vi "Execute_SQL.vi"(6 "commandTimeout in":i32=-1, 7 "CommandType":i32(ring)=-1 items=["Text"=1, "StoredProcedure"=4, "TableDirect"=512], 8 "error in (no error)":errorcluster, 9 "Parameters In":variant, 10 "sql":string, 11 "SqlMapper in":refnum<class "SqlMapper.lvclass">) -> (0 "error out":errorcluster, 1 "affectedRows":i32, 3 "SqlMapper out":refnum<class "SqlMapper.lvclass">)   [LabVIEW 2020, in "ORM_API.lvlib"]
uses:
  ORM_API.lvlib
  <vilib>/Viviota/shared/ORM.lvlibp/ORM/SqlMapper/SqlMapper.lvclass
  <vilib>/Viviota/shared/ORM.lvlibp/ORM/TypeMap/Create DynamicParameter.vi
  <vilib>/Viviota/shared/ORM.lvlibp/ORM/DynamicParameters/DynamicParameters.lvclass
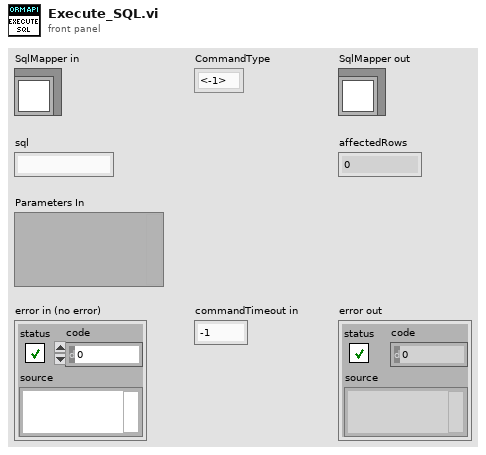
[diagram p1: front panel]
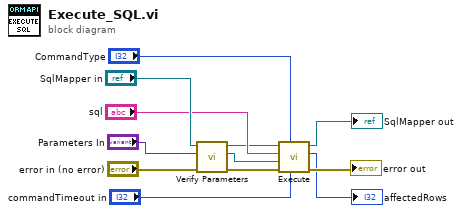
[diagram p0: block diagram]
diagram:
  n1 = call "Verify Parameters.vi"("error in (no error)"="error in (no error)", "Parameters In"="Parameters In", "SqlMapper in"="SqlMapper in") -> ("error out"=w7:errorcluster, "DynamicParameters out"=w6:refnum<class "DynamicParameters.lvclass">, "SqlMapper out"=w4:refnum<class "SqlMapper.lvclass">)  [unwired: 6 in]
  n2 = call-dynamic "Execute.vi"("commandTimeout"="commandTimeout in", "CommandType"="CommandType", "error in (no error)"=w7, "DynamicParameters"=w6, "sql"="sql", "SqlMapper in"=w4) -> ("error out"=→"error out":errorcluster, "affectedRows"=→"affectedRows":i32, "SqlMapper out"=→"SqlMapper out":refnum<class "SqlMapper.lvclass">)  [unwired: 3 in]
